vi "LinearSystemLoop_Reset.vi"(9 "initialState":T1, 11 "input inear System Loop":T2) -> (0 "Size Coerced":bool, 3 "out Linear System Loop":T2)   [LabVIEW 2019, in "Trajectory_Library.lvlib"]
doc: "Zeroes reference r and controller output u. The previous reference of the PlantInversionFeedforward and the initial state estimate of the KalmanFilter are set to the initial state provided.\n \nInputs:\n - LinearSystemLoop -- system data cluster\n - initialState -- The initial state.\n\nOutputs:\n - outLinearSystemLoop -- updated system data cluster\n - sizeCoerced -- If TRUE, an error occured."
uses:
  Trajectory_Library.lvlib
  TypeDef/LINEAR_SYSTEM_LOOP.ctl
  TypeDef/LINEAR_QUADRATIC_REGULATOR.ctl
  <vilib>/Analysis/Matrix/Datatypes/RealMatrix.ctl
  TypeDef/LINEAR_PLANT_INV_FF.ctl
  TypeDef/KALMAN_FILTER.ctl
  TypeDef/LINEAR_SYSTEM.ctl
  <vilib>/Analysis/Matrix/NI_Matrix.lvlib
panel:
  # "<States,1>"
  # "<FUTURE --- CLAMP TYPE -- For now\nuse Normalize>"
  # "Steady State Gain  \n<States,Outputs>"
  # "State Estimate <Statess,1>"
  # "<States,States>"
  # "<States,Inputs>"
  # "<Outputs,States>"
  # "<Outputs,Inputs>"
  # "<States,1>"
  # "<Inputs,1>"
  # "<States,Inputs>"
  # "<States,States>"
  # "Ref State <States,1>"
  # "Comp and capped \noutput <Inputs,1>"
  # "Controller gain\n<Inputs,States>"
  # "<States,1>"
  # "<FUTURE --- CLAMP TYPE -- For now\nuse Normalize>"
  # "Steady State Gain  \n<States,Outputs>"
  # "State Estimate <Statess,1>"
  # "<States,States>"
  # "<States,Inputs>"
  # "<Outputs,States>"
  # "<Outputs,Inputs>"
  # "<States,1>"
  # "<Inputs,1>"
  # "<States,Inputs>"
  # "<States,States>"
  # "Ref State <States,1>"
  # "Comp and capped \noutput <Inputs,1>"
  # "Controller gain\n<Inputs,States>"
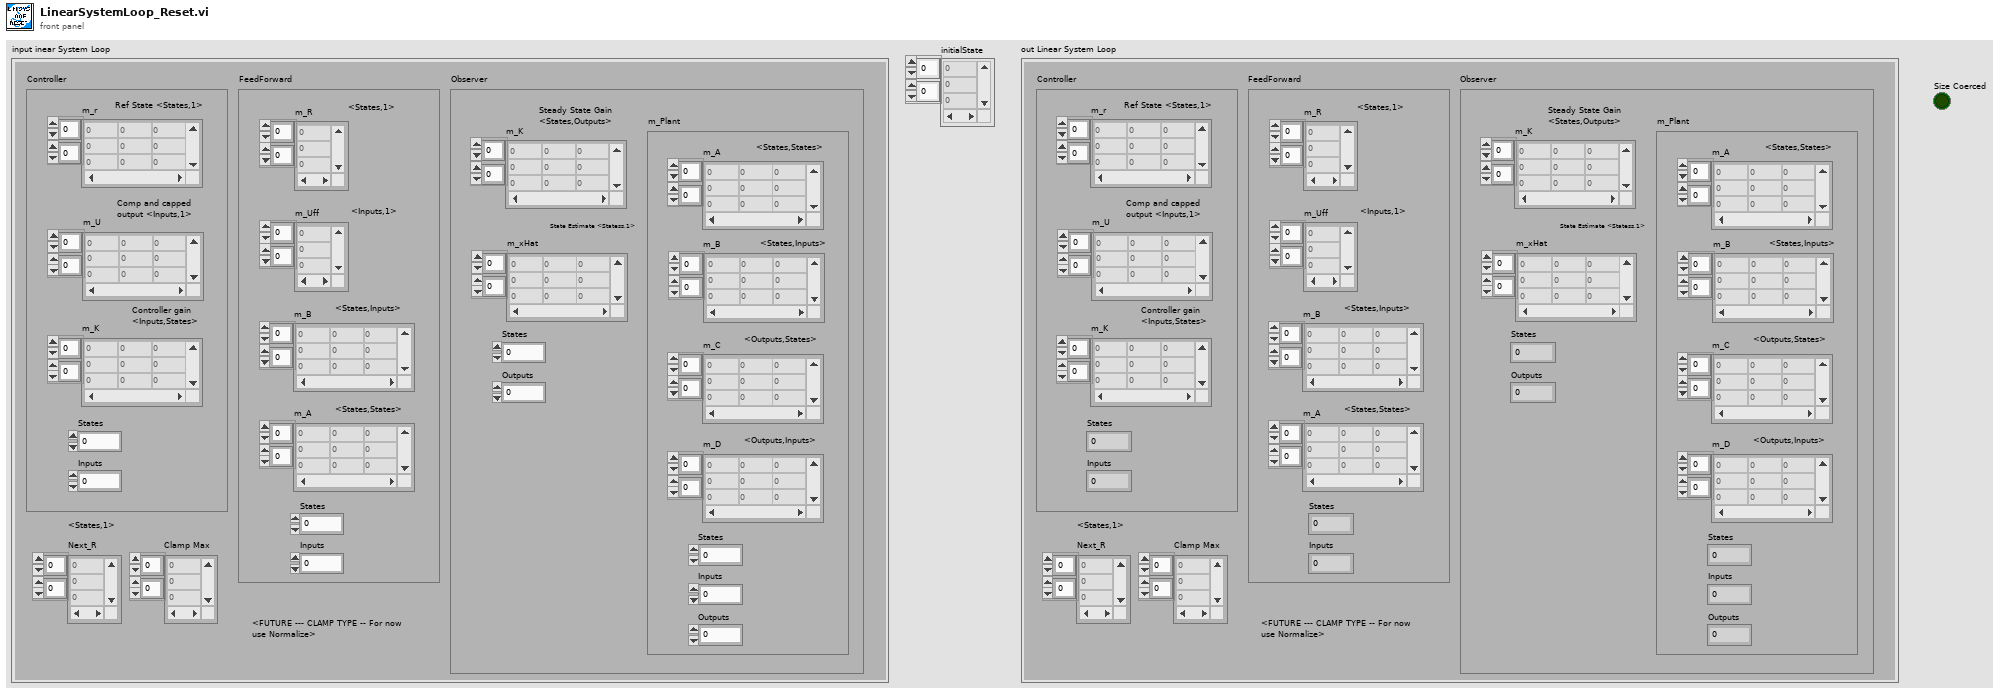
[diagram p1: front panel]
types:
  T1 = typedef "NI_Matrix.lvlib/RealMatrix.ctl" = dbl[][]
  T2 = typedef "Trajectory_Library.lvlib/LINEAR_SYSTEM_LOOP.ctl" = cluster{"Controller":T3, "FeedForward":T4, "Observer":T5, "Next_R":T1, "Clamp Max":T1}
  T3 = typedef "Trajectory_Library.lvlib/LINEAR_QUADRATIC_REGULATOR.ctl" = cluster{"m_r":T1, "m_U":T1, "m_K":T1, "States":i32, "Inputs":i32}
  T4 = typedef "Trajectory_Library.lvlib/LINEAR_PLANT_INV_FF.ctl" = cluster{"m_R":T1, "m_Uff":T1, "m_B":T1, "m_A":T1, "States":i32, "Inputs":i32}
  T5 = typedef "Trajectory_Library.lvlib/KALMAN_FILTER.ctl" = cluster{"m_K":T1, "m_xHat":T1, "States":i32, "Outputs":i32, "m_Plant":T6}
  T6 = typedef "Trajectory_Library.lvlib/LINEAR_SYSTEM.ctl" = cluster{"m_A":T1, "m_B":T1, "m_C":T1, "m_D":T1, "States":i32, "Inputs":i32, "Outputs":i32}
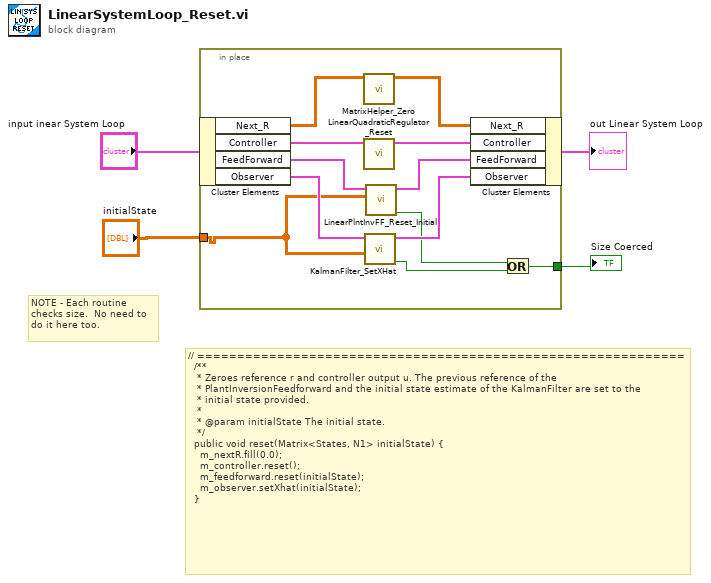
[diagram p0: block diagram]
diagram:
  # "NOTE - Each routine\nchecks size.  No need to\ndo it here too."
  # "// =============================================================\n  /**\n   * Zeroes reference r and controller output u. The previous reference of the\n   * PlantInversionFeedforward and the initial state estimate of the KalmanFilter are set to the\n   * initial state provided.\n   *\n   * @param initialState The initial state.\n   */\n  public void reset(Matrix<States, N1> initialState) {\n    m_nextR.fill(0.0);\n    m_controller.reset();\n    m_feedforward.reset(initialState);\n    m_observer.setXhat(initialState);\n  }"
  n1 = in-place {
    in-place-border: "initialState" -> [w12]
    in-place-border: [w5] -> w1
    n2 = in-place-cluster #1("input inear System Loop") -> ("Next_R"=w16:T1, "Controller"=w15:T3, "FeedForward"=w14:T4, "Observer"=w13:T5)
    n3 = call "MatrixHelper_Zero.vi"("input matrix"=w16) -> ("output matrix"=w11:T1)  [unwired: 10 in]
    n4 = call "LinearQuadraticRegulator_Reset.vi"("in LinearQuadraticRegulator"=w15) -> ("out LinearQuadraticRegulator"=w10:T3)  [unwired: 10 in]
    n5 = call "KalmanFilter_SetXHat.vi"("xHat"=w12, "in KalmanFilter"=w13) -> ("Size Coerced"=w6:bool, "out KalmanFilter"=w8:T5)  [unwired: 8 in]
    n6 = call "LinearPlntInvFF_Reset_Initial.vi"("initialState"=w12, "Input Linear Plant Inv FF"=w14) -> ("Size Coerced"=w7:bool, "Output Linear Plant Inv FF"=w9:T4)  [unwired: 8 in]
    n7 = in-place-cluster #1("Next_R"=w11, "Controller"=w10, "FeedForward"=w9, "Observer"=w8) -> (→"out Linear System Loop":T2)
    n8 = Or(x=w7, y=w6) -> (x .or. y?=w5:bool)
  }
  "Size Coerced" <- w1
